vi "Configure Session.vi"(4 "serialCfg":T1={"baud rate"=9600, "data bits"=7, "stop bits"=10, "parity"=2, "flow control"=0, "endModeforReads"=2, "endModeforWrites"=2} {"stop bits" items=["1.0"=10, "1.5"=15, "2.0"=20]; "parity" items=["None", "Odd", "Even", "Mark", "Space"]; "flow control" items=["None", "XON/XOFF", "RTS/CTS", "XON/XOFF & RTS/CTS", "DTR/DSR", "XON/XOFF & DTR/DSR"]; "endModeforReads" items=["None", "Last Bit", "TermChar"]; "endModeforWrites" items=["None", "Last Bit", "TermChar", "Break"]}, 6 "Message Cfg":T2={"sendEndEn"=TRUE, "suppEnEnRd"=FALSE, "termChar"=13, "EnTermChar"=TRUE}, 7 "timeout":u32=500, 8 "error in":errorcluster, 10 "VISA Resource":refnum<visa-resource-name>, 11 "Serial Session":refnum<class "Serial Session.lvclass">) -> (0 "error out":errorcluster, 3 "Serial Session out":refnum<class "Serial Session.lvclass">)   [LabVIEW 2015, in "Serial Session.lvclass"]
doc: "Configures a session using the VISA serial property nodes. Call this before opening any references to the session. After this, the ESF will handle all calls to the port via the session handle."
uses:
  Serial Session.lvclass
  Typedefs/Msg Config.ctl
  Typedefs/Serial Config.ctl
  Serial Session.lvclass/Serial Session.ctl
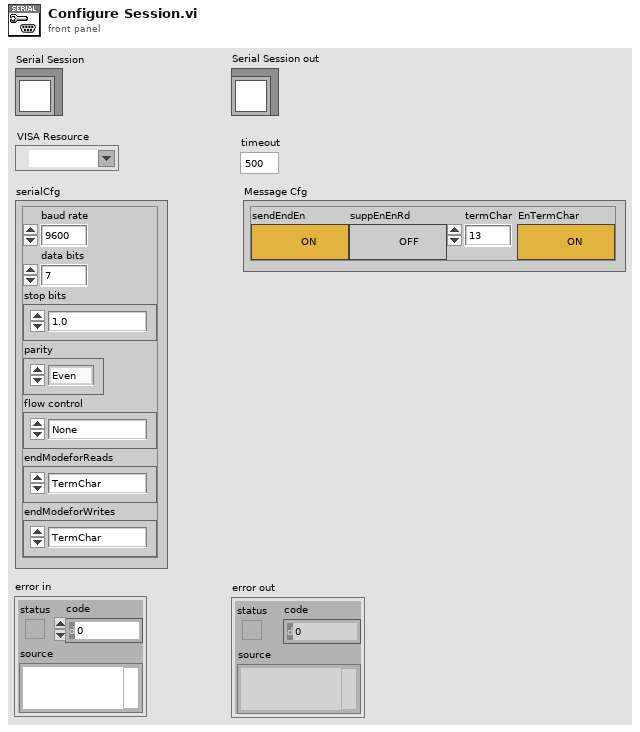
[diagram p1: front panel]
types:
  T1 = typedef "Serial Session.lvclass/Serial Config.ctl" = cluster{"baud rate":u32, "data bits":u16, "stop bits":u16, "parity":u16, "flow control":u16, "endModeforReads":u16, "endModeforWrites":u16}
  T2 = typedef "Serial Session.lvclass/Msg Config.ctl" = cluster{"sendEndEn":bool, "suppEnEnRd":bool, "termChar":u8, "EnTermChar":bool}
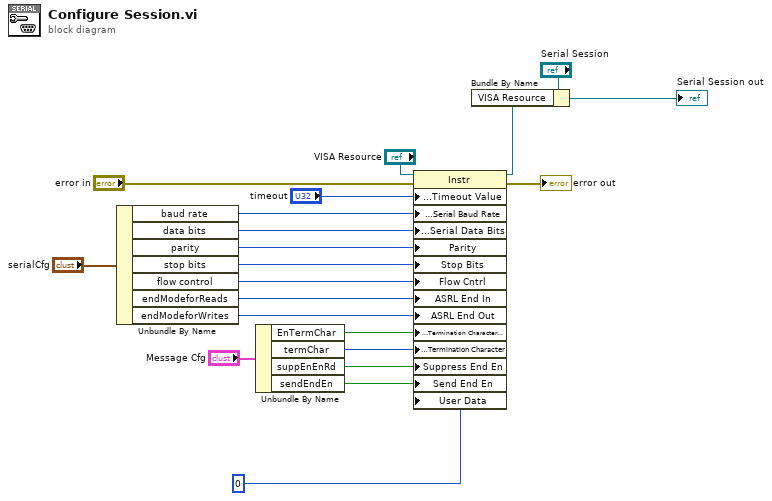
[diagram p0: block diagram]
diagram:
  n1 = Unbundle By Name("serialCfg") -> ("baud rate"=w20:u32, "data bits"=w19:u16, "parity"=w18:u16, "stop bits"=w17:u16, "flow control"=w16:u16, "endModeforReads"=w15:u16, "endModeforWrites"=w14:u16)
  n2 = Unbundle By Name("Message Cfg") -> ("EnTermChar"=w13:bool, "termChar"=w12:u8, "suppEnEnRd"=w11:bool, "sendEndEn"=w10:bool)
  n3 = property class="Instr"(reference="VISA Resource", error in="error in", "General Settings:Timeout Value"="timeout", "Serial Settings:Serial Baud Rate"=w20, "Serial Settings:Serial Data Bits"=w19, "Parity"=w18, "Stop Bits"=w17, "Flow Cntrl"=w16, "ASRL End In"=w15, "ASRL End Out"=w14, "Message Based Settings:Termination Character Enable"=w13, "Message Based Settings:Termination Character"=w12, "Suppress End En"=w11, "Send End En"=w10, "User Data"=u32 0 ("General Settings:User Data")) -> (reference out=w7:refnum<visa-resource-name>, error out=→"error out":errorcluster)
  n4 = Bundle By Name(cluster="Serial Session", "VISA Resource"=w7) -> (→"Serial Session out":refnum<class "Serial Session.lvclass">)
